vi "omni drive.vi"(0 "Drive RefNum":T3={"DevStatus"={"status"=FALSE, "code"=0, "source"=""}, "Motors[]"=[], "Square Inputs"=FALSE, "Max Output"=1.0}, 1 "X Axis":dbl, 2 "Y Axis":dbl, 3 "Z Axis":dbl, 4 "Drive Mode":T1=enum."Arcade Drive", 5 "Center Motor":T4={"DeviceStatus"={"status"=FALSE, "code"=0, "source"=""}, "Type"=enum."PWM", "PWM"={"Controller"=enum."Controller 1", "PWM Channel"=enum."Invalid", "DeadBand"={"Name"="", "maxPositivePwm"=0, "minPositivePwm"=0, "centerPwm"=0, "maxNegativePwm"=0, "minNegativePwm"=0, "angularRange"=0}}, "CAN"={"Device Number"=0, "Control Mode"=enum."Percent VBus", "Semaphore"=refnum, "Max Vout"=12.0, "TalonSRX Control Mode"=enum."Percent VBus"}, "Invert"=FALSE, "TransformRef"=refnum, "InvTransformRef"=refnum}) -> ()   [LabVIEW 2014]
uses:
  typedefs/omni drive mode.ctl
  <vilib>/Rock Robotics/WPI/RobotDrive/WPI_RobotDriveDevRef.ctl
  <vilib>/Rock Robotics/WPI/MotorControl/WPI_MotorControlDeviceRef.ctl
  <vilib>/Rock Robotics/WPI/MotorControl/WPI_MotorControlType.ctl
  <vilib>/Rock Robotics/SystemInterfaces/Typedef/FPGA_TypedefDigitalModule.ctl
  <vilib>/Rock Robotics/SystemInterfaces/DIO/FPGA_DIOPWMChannel.ctl
  <vilib>/Rock Robotics/WPI/PWM/WPI_PWMDeadband.ctl
  <vilib>/Rock Robotics/WPI/CAN/Jaguar/SubVIs/WPI_CANJaguar_ControlMode.ctl
  <vilib>/Rock Robotics/WPI/CAN/TalonSRX/WPI_CANTalonSRX_APIControlMode.ctl
  <vilib>/Rock Robotics/WPI/PWM/WPI_PWMTransform_ConPane.ctl
  global variables/devrefs.vi
  <vilib>/addons/control/pid/pid.llb/PID (DBL).vi
  <vilib>/Rock Robotics/WPI/RobotDrive/WPI_RobotDriveArcadeDrive_Standard(NoSaturation).vi
  global variables/dashboard data.vi
  <vilib>/addons/control/pid/NI_PID_pid.lvlib
panel:
  in  "Omni-Drive Tab Control":enum32{"Drive I/O", "PID", "Motor Controls"}(tab)
  in  "Spin Factor":dbl(slide) min=0.0 max=2.0 step=0.1 scale=0.0..2.0
  in  "PID Gains":T2={"proportional gain (Kc)"=0.003, "integral time (Ti, min)"=0.0012, "derivative time (Td, min)"=0.001} {"derivative time (Td, min)" step=0.0001 format="%.5f"; "integral time (Ti, min)" step=0.0001 format="%.5f"; "proportional gain (Kc)" step=0.0001 format="%.5f"}
  out "Gyro Temp °C":dbl
  out "Gyro Temp °F":dbl
  out "Setpoint Angle":dbl format="%#_6g°"
  out "Current Angle":dbl format="%#_g°"
  out "PID & Gyro Waveform Chart":cluster{"Angle":dbl, "output":dbl}(graph)
  out "Angular Rate":dbl
  # "Drive the Robot in Either Arcade Style or H-Drive Style"
  # "VI Inputs"
  # "OKish values rev1\nP: 0.00040\nI: 0.00100\nD: 0.00000\n\nPretty Good values\nP: 0.02\nI: 0.005\nD: 0.001\n\nBetter values?\nP: 0.0025\nI: 0.002\nD: 0.001"
  # "Thats a type def so you can't change it to the system\ncontrol otherwise it will no longer by linked to the typedef,\nand you can't re-link it"
  # "Temporary"
  # "Does this empty space make you feel uncomfortable?"
  # "Yes."
  # "I'm glad you feel that way."
  # "Note: Current Angle only updated in H-Drive, \nSetpoint updated in Arcade"
  # "°/sec"
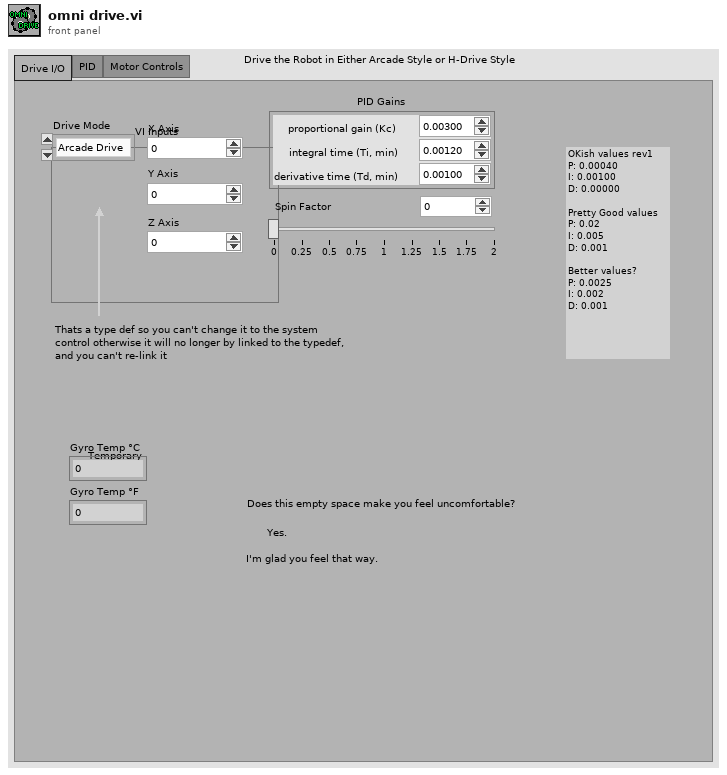
[diagram p1: front panel]
types:
  T1 = typedef "omni drive mode.ctl" = enum16{"Left/Right X/Y Control", "Arcade Drive", "H-Drive", "H-Drive Spin", "H-Drive PID", "Autonomous"}
  T2 = cluster{"proportional gain (Kc)":dbl, "integral time (Ti, min)":dbl, "derivative time (Td, min)":dbl}
  T3 = typedef "WPI_RobotDriveDevRef.ctl" = cluster{"DevStatus":errorcluster, "Motors[]":T4[], "Square Inputs":bool, "Max Output":dbl}
  T4 = typedef "WPI_MotorControlDeviceRef.ctl" = cluster{"DeviceStatus":errorcluster, "Type":T5, "PWM":cluster{"Controller":T6, "PWM Channel":T7, "DeadBand":T8}, "CAN":cluster{"Device Number":u8, "Control Mode":T9, "Semaphore":T10, "Max Vout":dbl, "TalonSRX Control Mode":T11}, "Invert":bool, "TransformRef":T12, "InvTransformRef":T12}
  T5 = typedef "WPI_MotorControlType.ctl" = enum16{"PWM", "CAN", "CANTalonSRX"}
  T6 = typedef "FPGA_TypedefDigitalModule.ctl" = enum16{"Controller 1"}
  T7 = typedef "FPGA_DIOPWMChannel.ctl" = enum8{"PWM 0", "PWM 1", "PWM 2", "PWM 3", "PWM 4", "PWM 5", "PWM 6", "PWM 7", "PWM 8", "PWM 9", "PWM MXP 0", "PWM MXP 1", "PWM MXP 2", "PWM MXP 3", "PWM MXP 4", "PWM MXP 5", "PWM MXP 6", "PWM MXP 7", "PWM MXP 8", "PWM MXP 9", "Invalid"}
  T8 = typedef "WPI_PWMDeadband.ctl" = cluster{"Name":string, "maxPositivePwm":i32, "minPositivePwm":i32, "centerPwm":i32, "maxNegativePwm":i32, "minNegativePwm":i32, "angularRange":u16}
  T9 = typedef "WPI_CANJaguar_ControlMode.ctl" = enum8{"Percent VBus", "Current", "Speed", "Position", "Voltage"}
  T10 = typedef "Semaphore RefNum" = refnum<k1>
  T11 = typedef "WPI_CANTalonSRX_APIControlMode.ctl" = enum8{"Percent VBus", "Speed", "Position", "Slave", "Unchanged / Invalid"}
  T12 = typedef "WPI_PWMTransform_ConPane.ctl" = refnum<vi>
  T13 = typedef "WPI_GyroDevRef.ctl" = cluster{"DevStatus":errorcluster, "Analog Module":T14, "Analog Channel":T15, "Offset":dbl, "Gain (VoltsPerDegree/Second)":dbl}
  T14 = typedef "FPGA_TypedefAnalogModule.ctl" = enum16{"Controller 1"}
  T15 = typedef "FPGA_AIChannel.ctl" = enum8{"AI 0", "AI 1", "AI 2", "AI 3", "AI MXP 0", "AI MXP 1", "AI MXP 2", "AI MXP 3", "Invalid"}
  T16 = typedef "WPI_EncoderDevRef.ctl" = cluster{"DevStatus":errorcluster, "EncoderIndex":T17, "CounterIndex":T18, "DistancePerCount":dbl, "Decoding Type":T19}
  T17 = typedef "FPGA_EncoderIdx.ctl" = enum8{"Enc 0", "Enc 1", "Enc 2", "Enc 3", "Enc 4", "Enc 5", "Enc 6", "Enc 7", "Invalid"}
  T18 = typedef "FPGA_CounterCtrSystemIndex.ctl" = enum8{"Ctr 0", "Ctr 1", "Ctr 2", "Ctr 3", "Ctr 4", "Ctr 5", "Ctr 6", "Ctr 7", "Invalid"}
  T19 = typedef "WPI_EncoderType.ctl" = enum16{"1x", "2x", "4x"}
  T20 = typedef "WPI_AnalogChannelDevRef.ctl" = cluster{"DevStatus":errorcluster, "Controller":T14, "Analog Channel":T15}
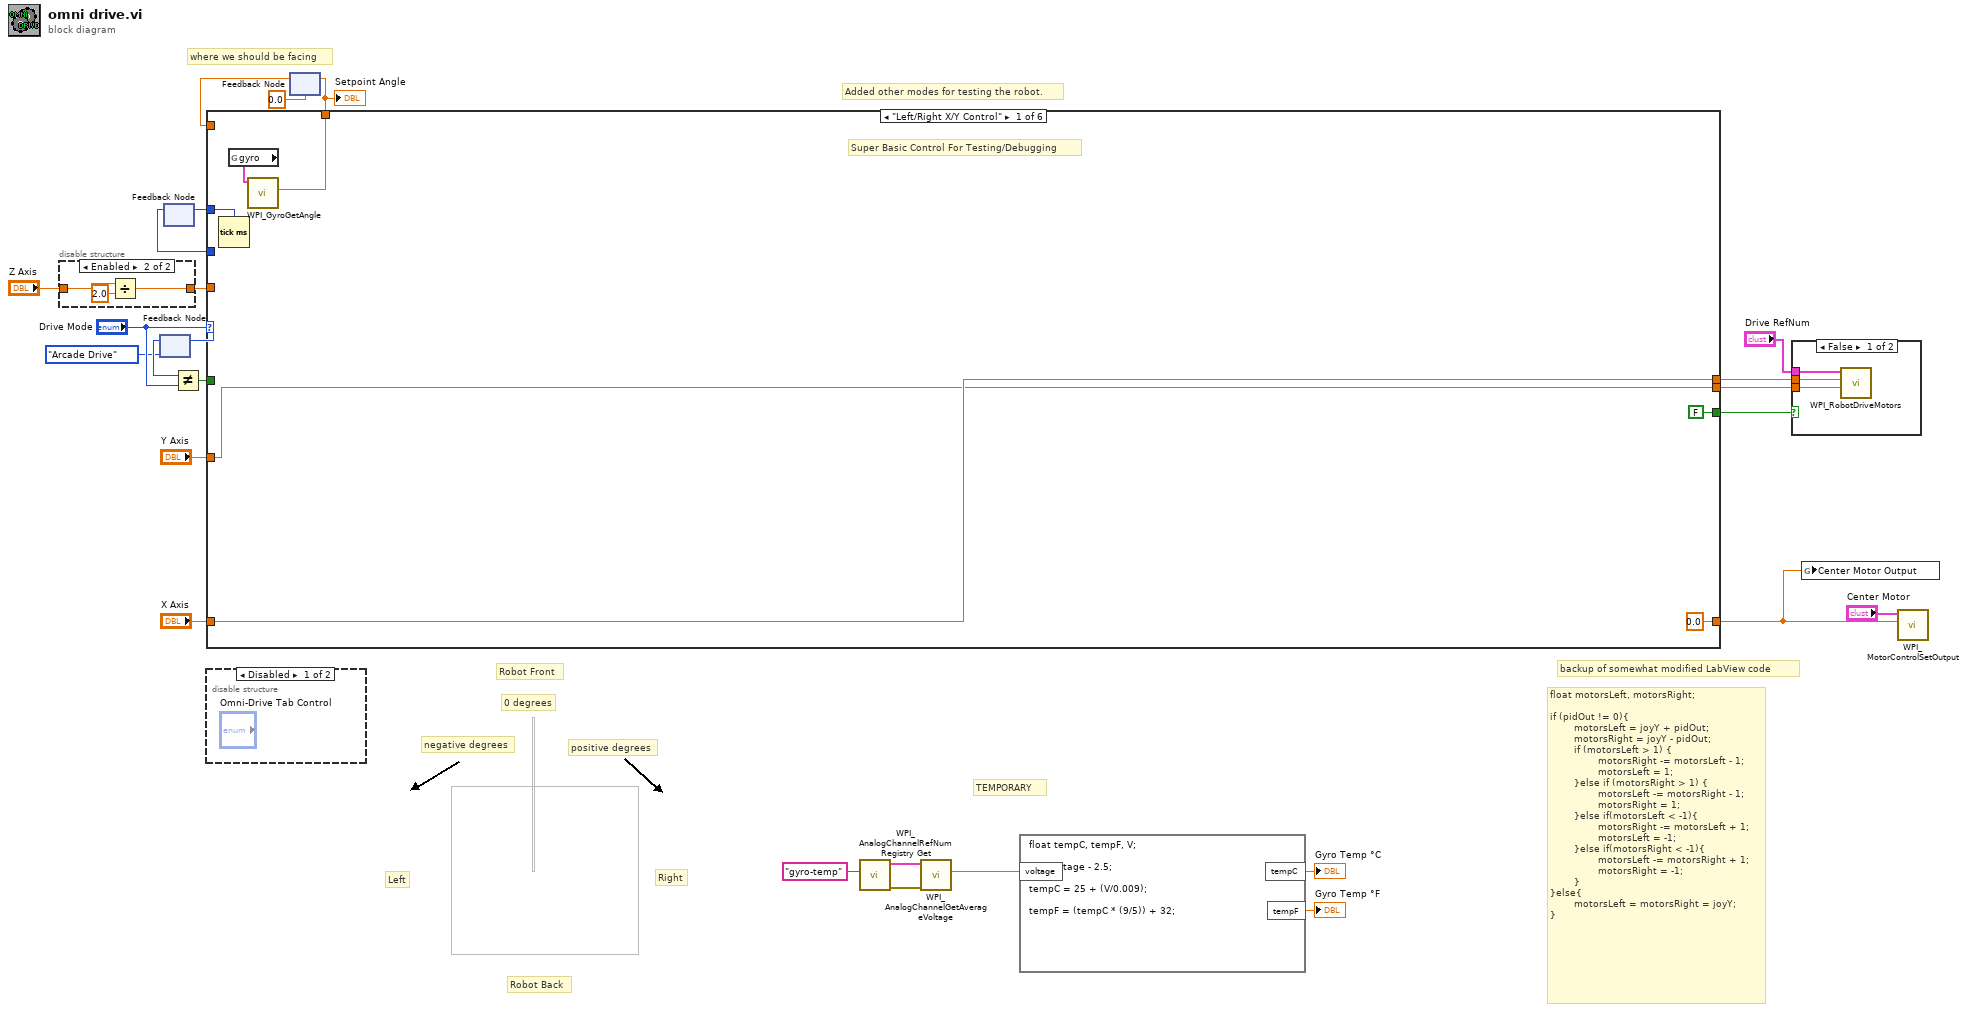
[diagram p0: block diagram]
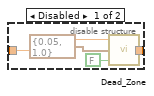
[diagram p2: hidden frame]
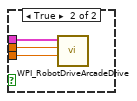
[diagram p4: hidden frame]
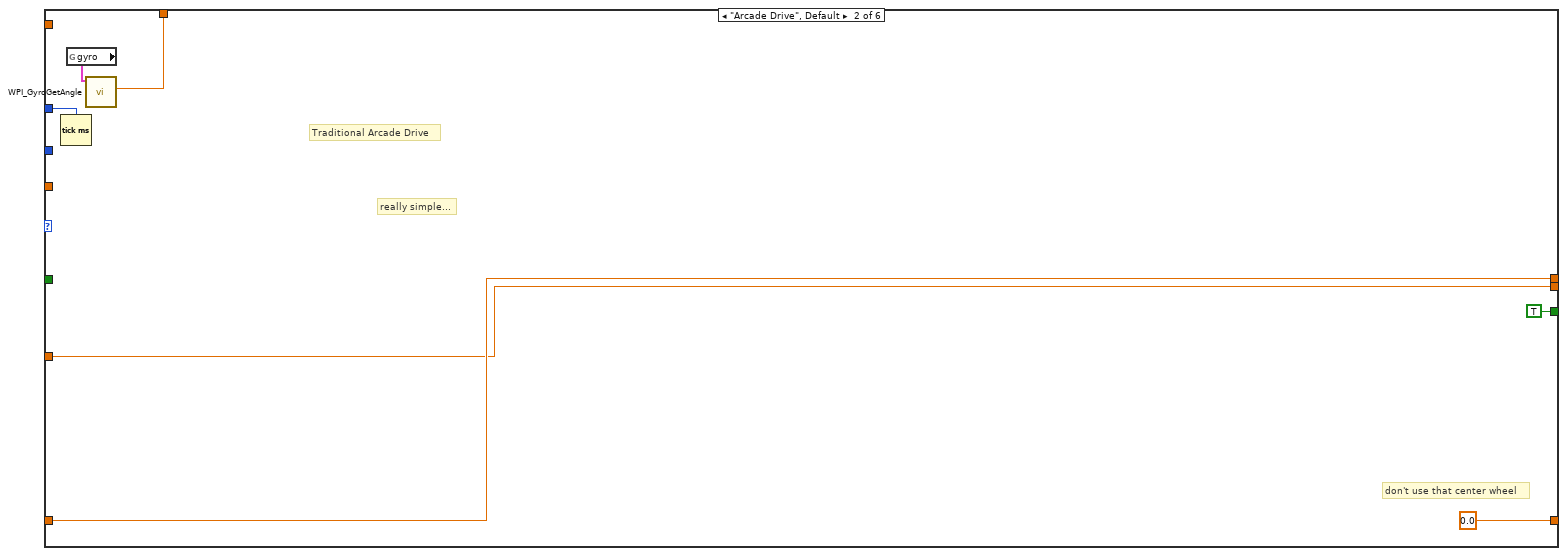
[diagram p5: hidden frame]
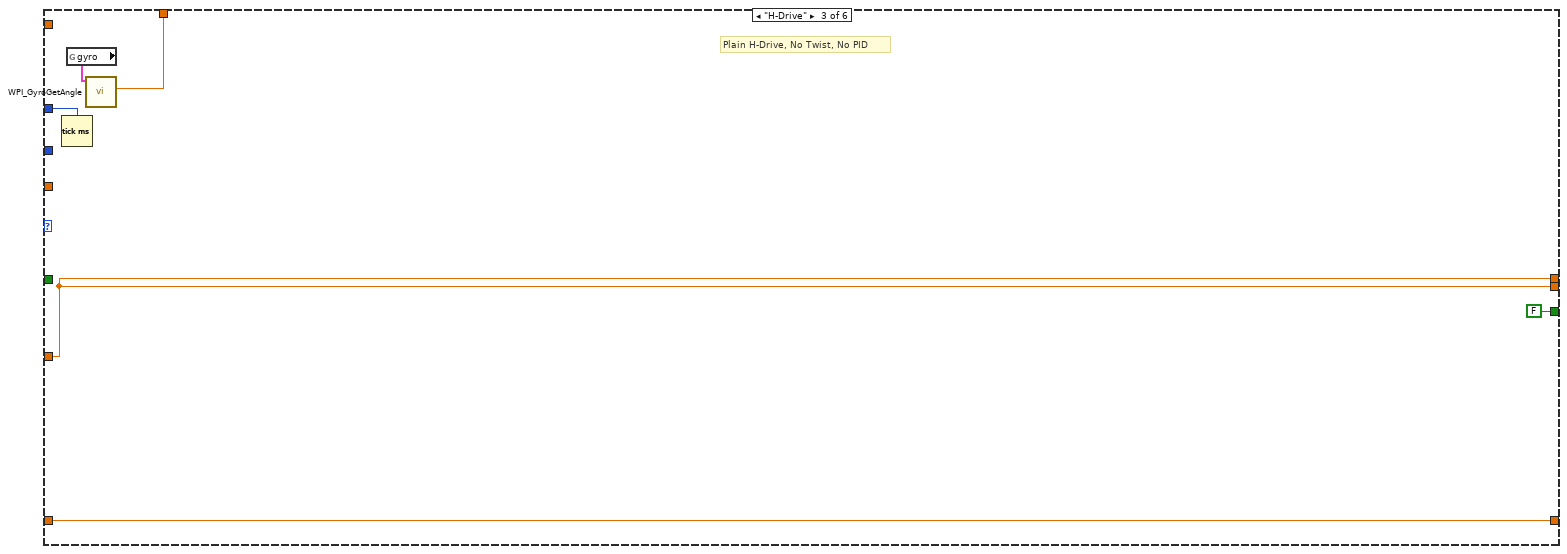
[diagram p6: hidden frame]
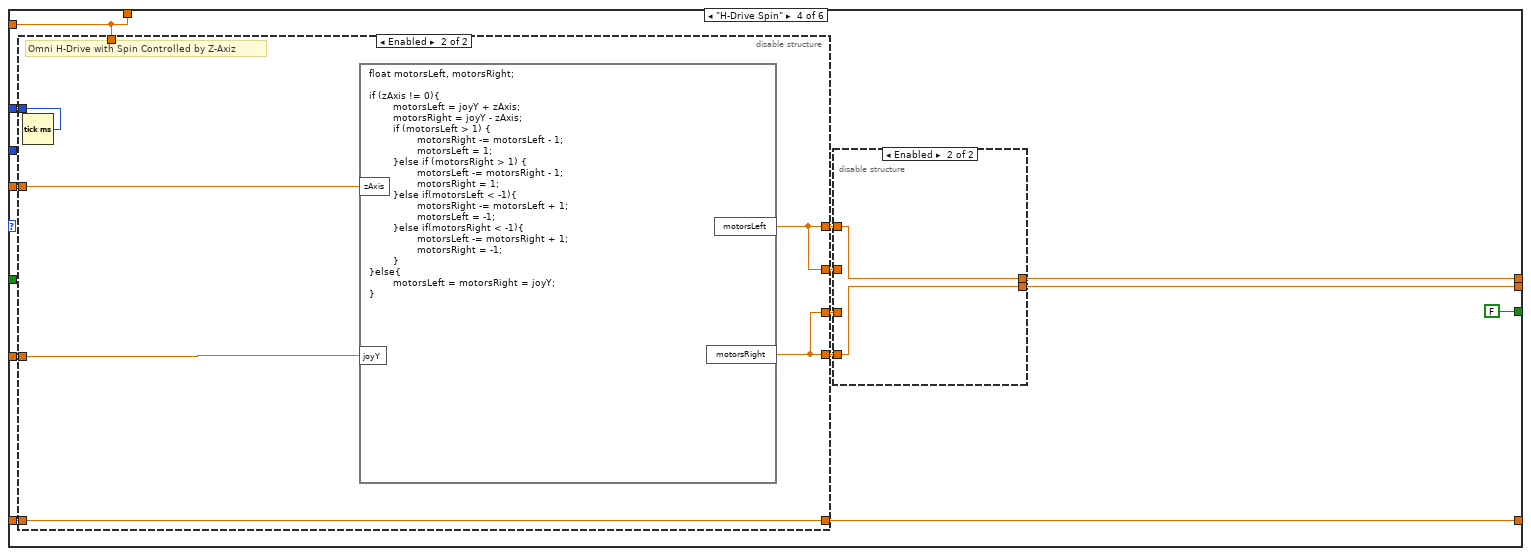
[diagram p7: hidden frame]
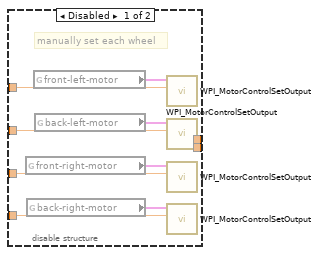
[diagram p8: hidden frame]
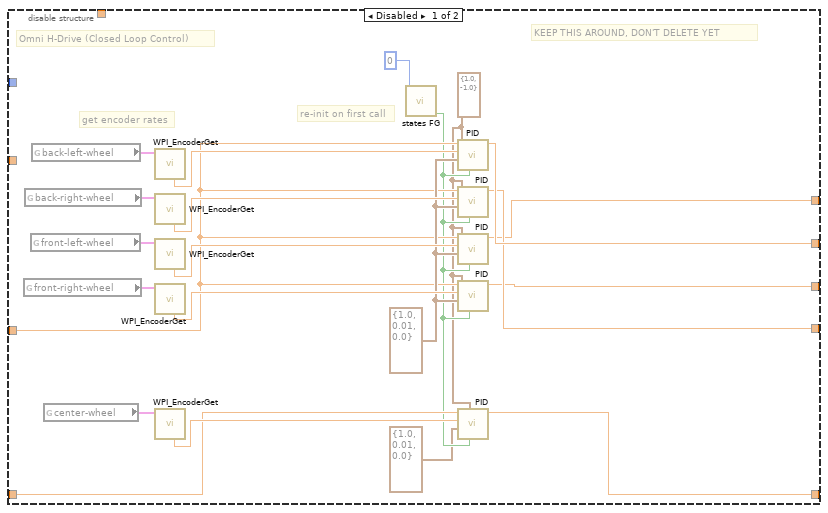
[diagram p9: hidden frame]
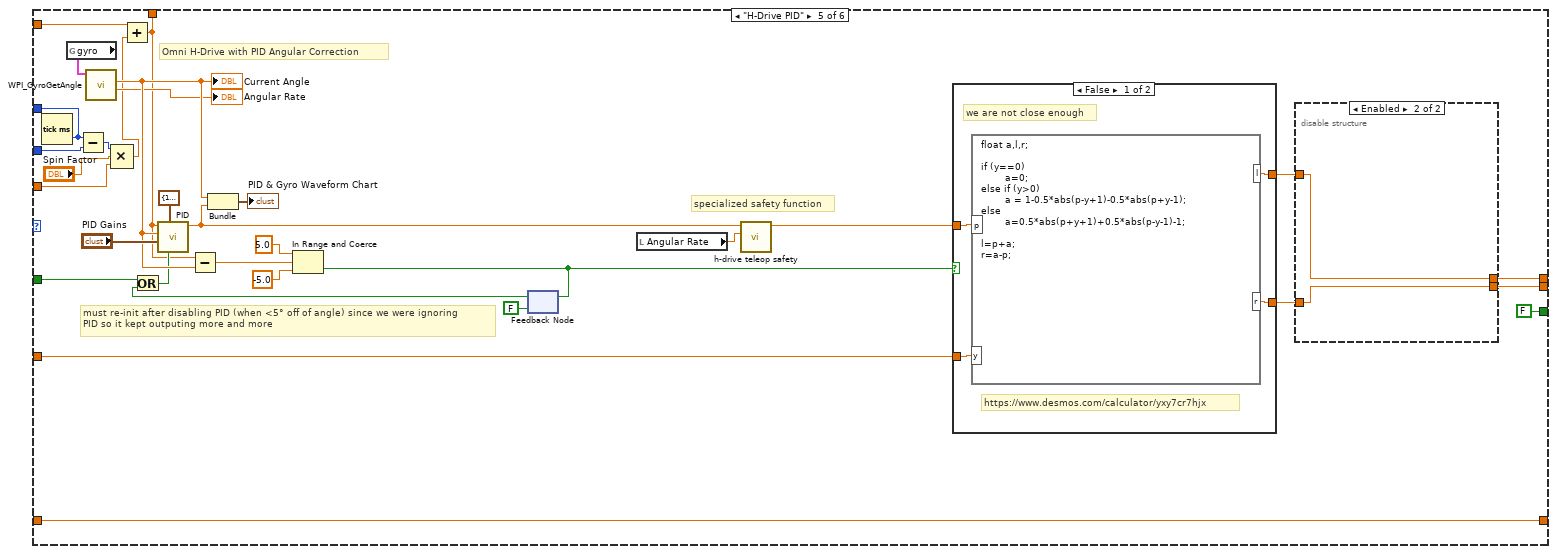
[diagram p10: hidden frame]
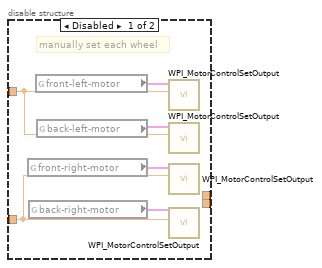
[diagram p11: hidden frame]
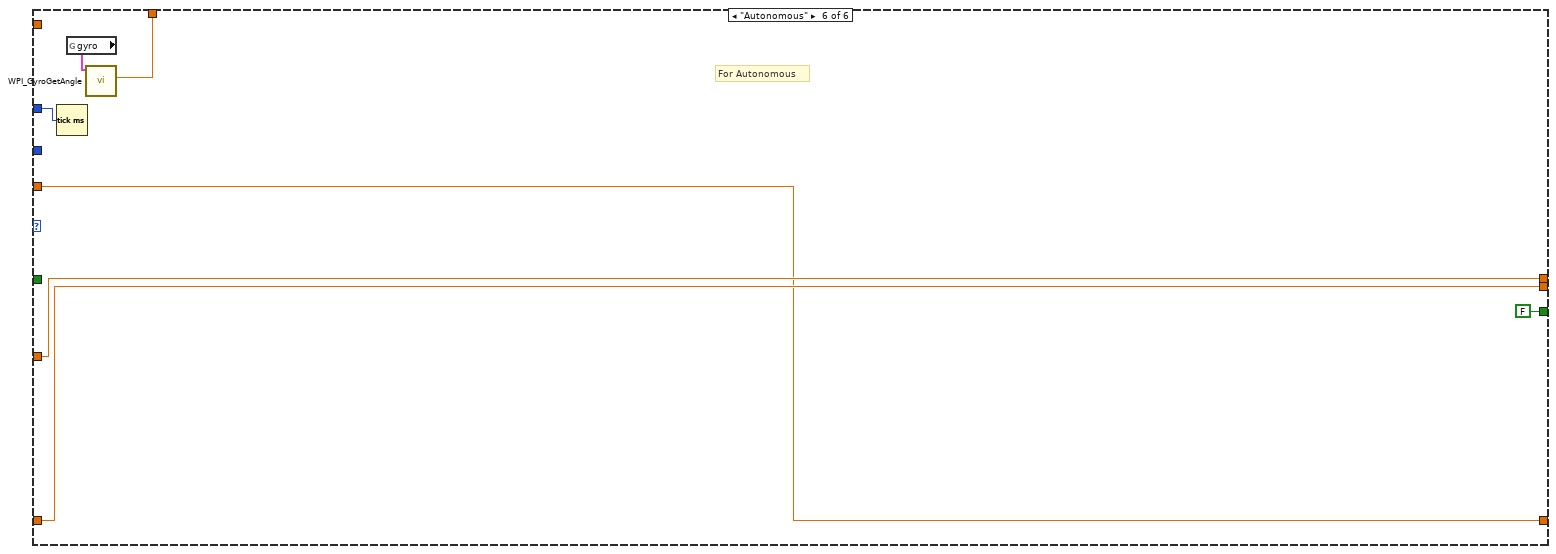
[diagram p13: hidden frame]
diagram:
  # "Added other modes for testing the robot."
  # "TEMPORARY"
  # "backup of somewhat modified LabView code"
  # "float motorsLeft, motorsRight;\n\nif (pidOut != 0){\n        motorsLeft = joyY + pidOut;\n        motorsRight = joyY - pidOut;\n        if (motorsLeft > 1) {\n                motorsRight -= motorsLeft - 1;\n                motorsLeft = 1;\n        }else if (motorsRight > 1) {\n                motorsLeft -= motorsRight - 1;\n                motorsRight = 1;\n        }else if(motorsLeft < -1){\n                motorsRight -= motorsLeft + 1;\n                motorsLeft = -1;\n        }else if(motorsRight < -1){\n                motorsLeft -= motorsRight + 1;\n                motorsRight = -1;\n        }\n}else{\n        motorsLeft = motorsRight = joyY;\n}"
  # "Robot Back"
  # "Right"
  # "Left"
  # "negative degrees"
  # "positive degrees"
  # "0 degrees"
  # "Robot Front"
  # "where we should be facing"
  n1 = disable-structure shown="Enabled" {
    disable-tunnel: [w29 w32] -> w2
    disable-tunnel: "Z Axis" -> [w28 w31]
    frame Disabled {
      n2 = call "Dead_Zone.vi"("Slope of 1"=FALSE, "Dead Zone and Limits"=cluster{dbl, dbl} {0.05, 1.0}, "Input"=w28) -> ("Output"=w29:dbl)  [unwired: 1 in]
    }
    frame Enabled {
      n3 = Divide(x=w31, y=2.0) -> (x/y=w32:dbl)
    }
  }
  n4 = feedback-in #1("Drive Mode") -> ()
  n5 = feedback #1(omni_drive_mode."Arcade Drive" ("Drive Mode")) -> (w18:T1)
  n6 = feedback #2() -> (w3:u32)  [unwired: 1 in]
  n7 = Not Equal?(x=w18, y="Drive Mode") -> (x != y?=w16:bool)
  n8 = disable-structure shown="Disabled" {
    frame Disabled {
    }
    frame Enabled {
    }
  }
  n9 = feedback #3(0.0) -> (w5:dbl)
  n10 = case shown="\"Left/Right X/Y Control\"" "Drive Mode" {
    tunnel: [0.0 ("X Axis") 0.0 w50 w62 w133 w152] -> w6
    tunnel: [w38 w45 w51 w54 w112 w153] -> w25
    tunnel: [w39 w46 w51 w55 w113 w155] -> w24
    tunnel: "X Axis" -> [w39 w46 w50 w63 w133 w153]
    tunnel: "Y Axis" -> [w38 w45 w51 w64 w134 w155]
    tunnel: [FALSE TRUE FALSE FALSE FALSE FALSE] -> w21
    tunnel: w16 -> [_ _ _ _ w132 _]
    tunnel: [w34 w43 w48 w61 w105 w150] -> w15
    tunnel: w5 -> [_ _ _ w61 w106 _]
    tunnel: w2 -> [_ _ _ w56 w108 w152]
    tunnel: [w33 w40 w47 w53 w111 w149] -> w4
    tunnel: w3 -> [_ _ _ _ w110 _]
    frame "Left/Right X/Y Control" {
      # "Super Basic Control For Testing/Debugging"
      n11 = Tick Count (ms)() -> (millisecond timer value=w33:u32)
      n12 = global read "devrefs.vi" "gyro"() -> (w35:T13)
      n13 = call <vilib>:"WPI_GyroGetAngle.vi"("GyroDevRef"=w35) -> ("Angle"=w34:dbl)  [unwired: 7 in, 3 out]
    }
    frame "Arcade Drive", Default {
      # "really simple..."
      # "don't use that center wheel"
      # "Traditional Arcade Drive"
      n14 = Tick Count (ms)() -> (millisecond timer value=w40:u32)
      n15 = global read "devrefs.vi" "gyro"() -> (w44:T13)
      n16 = call <vilib>:"WPI_GyroGetAngle.vi"("GyroDevRef"=w44) -> ("Angle"=w43:dbl)  [unwired: 7 in, 3 out]
    }
    frame "H-Drive" {
      # "Plain H-Drive, No Twist, No PID"
      n17 = Tick Count (ms)() -> (millisecond timer value=w47:u32)
      n18 = global read "devrefs.vi" "gyro"() -> (w49:T13)
      n19 = call <vilib>:"WPI_GyroGetAngle.vi"("GyroDevRef"=w49) -> ("Angle"=w48:dbl)  [unwired: 7 in, 3 out]
    }
    frame "H-Drive Spin" {
      n20 = disable-structure shown="Enabled" {
        disable-tunnel: w64 -> [w86 w103]
        disable-tunnel: w63 -> [w84 w102]
        disable-tunnel: [w80 w102] -> w62
        disable-tunnel: w61 -> [_ _]
        disable-tunnel: [w77 w101] -> w60
        disable-tunnel: [w79 w101] -> w59
        disable-tunnel: [w78 w100] -> w57
        disable-tunnel: [w76 w100] -> w58
        disable-tunnel: w56 -> [_ w98]
        disable-tunnel: [_ w99] -> w53
        frame Disabled {
          w87 = T2 {"proportional gain (Kc)"=1.0, "integral time (Ti, min)"=0.01, "derivative time (Td, min)"=0.0} ("PID gains")
          w82 = cluster{"output high":dbl, "output low":dbl} {"output high"=1.0, "output low"=-1.0} ("output range")
          # "KEEP THIS AROUND, DON'T DELETE YET"
          # "re-init on first call"
          # "get encoder rates"
          # "Omni H-Drive (Closed Loop Control)"
          n21 = global read "devrefs.vi" "front-right-wheel"() -> (w94:T16)
          n22 = global read "devrefs.vi" "back-right-wheel"() -> (w96:T16)
          n23 = global read "devrefs.vi" "front-left-wheel"() -> (w95:T16)
          n24 = global read "devrefs.vi" "back-left-wheel"() -> (w97:T16)
          n25 = global read "devrefs.vi" "center-wheel"() -> (w93:T16)
          n26 = call <vilib>:"WPI_EncoderGet.vi"("EncoderDevRef"=w97) -> ("Rate"=w91:dbl)  [unwired: 5 in, 5 out]
          n27 = call <vilib>:"WPI_EncoderGet.vi"("EncoderDevRef"=w96) -> ("Rate"=w90:dbl)  [unwired: 5 in, 5 out]
          n28 = call <vilib>:"WPI_EncoderGet.vi"("EncoderDevRef"=w95) -> ("Rate"=w89:dbl)  [unwired: 5 in, 5 out]
          n29 = call <vilib>:"WPI_EncoderGet.vi"("EncoderDevRef"=w94) -> ("Rate"=w88:dbl)  [unwired: 5 in, 5 out]
          n30 = call <vilib>:"WPI_EncoderGet.vi"("EncoderDevRef"=w93) -> ("Rate"=w85:dbl)  [unwired: 5 in, 5 out]
          n31 = call "states FG.vi"("Loop ID"=0) -> ("first call?"=w83:bool)  [unwired: 7 in, 3 out]
          n32 = call-poly <vilib>:"PID.vi"("reinitialize? (F)"=w83, "output range"=w82, "PID gains"=w87, "process variable"=w91, "setpoint"=w86) -> ("output"=w79:dbl)  [unwired: 5 in, 1 out]
          n33 = call-poly <vilib>:"PID.vi"("reinitialize? (F)"=w83, "output range"=w82, "PID gains"=w87, "process variable"=w90, "setpoint"=w86) -> ("output"=w78:dbl)  [unwired: 5 in, 1 out]
          n34 = call-poly <vilib>:"PID.vi"("reinitialize? (F)"=w83, "output range"=w82, "PID gains"=w87, "process variable"=w89, "setpoint"=w86) -> ("output"=w77:dbl)  [unwired: 5 in, 1 out]
          n35 = call-poly <vilib>:"PID.vi"("reinitialize? (F)"=w83, "output range"=w82, "PID gains"=w87, "process variable"=w88, "setpoint"=w86) -> ("output"=w76:dbl)  [unwired: 5 in, 1 out]
          n36 = call-poly <vilib>:"PID.vi"("reinitialize? (F)"=w83, "output range"=w82, "PID gains"=T2 {"proportional gain (Kc)"=1.0, "integral time (Ti, min)"=0.01, "derivative time (Td, min)"=0.0}, "process variable"=w85, "setpoint"=w84) -> ("output"=w80:dbl)  [unwired: 5 in, 1 out]
        }
        frame Enabled {
          # "Omni H-Drive with Spin Controlled by Z-Axiz"
          n37 = Tick Count (ms)() -> (millisecond timer value=w99:u32)
          n38 = formula code="float motorsLeft, motorsRight;\n\nif (zAxis != 0){\n        motorsLeft = joyY + zAxis;\n        motorsRight = joyY - zAxis;\n        if (motorsLeft > 1) {\n                motorsRight -= motorsLeft - 1;\n                motorsLeft = 1;\n        }else if (motorsRight > 1) {\n                motorsLeft -= motorsRight - 1;\n                motorsRight = 1;\n        }else if(motorsLeft < -1){\n                motorsRight -= motorsLeft + 1;\n                motorsLeft = -1;\n        }else if(motorsRight < -1){\n                motorsLeft -= motorsRight + 1;\n                motorsRight = -1;\n        }\n}else{\n        motorsLeft = motorsRight = joyY;\n}"("zAxis"=w98, "joyY"=w103) -> ("motorsLeft"=w101:dbl, "motorsRight"=w100:dbl)
        }
      }
      n39 = disable-structure shown="Enabled" {
        disable-tunnel: w60 -> [w69 w75]
        disable-tunnel: w59 -> [w68 _]
        disable-tunnel: w58 -> [w67 _]
        disable-tunnel: w57 -> [w66 w74]
        disable-tunnel: [_ w75] -> w55
        disable-tunnel: [_ w74] -> w54
        frame Disabled {
          # "manually set each wheel"
          n40 = global read "devrefs.vi" "front-right-motor"() -> (w70:T4)
          n41 = global read "devrefs.vi" "back-right-motor"() -> (w72:T4)
          n42 = global read "devrefs.vi" "front-left-motor"() -> (w71:T4)
          n43 = global read "devrefs.vi" "back-left-motor"() -> (w73:T4)
          n44 = call <vilib>:"WPI_MotorControlSetOutput.vi"("Output"=w69, "MotorControlDevRef"=w71) -> ()  [unwired: 7 in, 3 out]
          n45 = call <vilib>:"WPI_MotorControlSetOutput.vi"("Output"=w68, "MotorControlDevRef"=w73) -> ()  [unwired: 7 in, 3 out]
          n46 = call <vilib>:"WPI_MotorControlSetOutput.vi"("Output"=w67, "MotorControlDevRef"=w70) -> ()  [unwired: 7 in, 3 out]
          n47 = call <vilib>:"WPI_MotorControlSetOutput.vi"("Output"=w66, "MotorControlDevRef"=w72) -> ()  [unwired: 7 in, 3 out]
        }
        frame Enabled {
        }
      }
    }
    frame "H-Drive PID" {
      # "specialized safety function"
      # "must re-init after disabling PID (when <5° off of angle) since we were ignoring\nPID so it kept outputing more and more"
      # "Omni H-Drive with PID Angular Correction"
      n48 = Tick Count (ms)() -> (millisecond timer value=w111:u32)
      n49 = global read "devrefs.vi" "gyro"() -> (w128:T13)
      n50 = Subtract(x=w111, y=w110) -> (x-y=w109:u32)
      n51 = call <vilib>:"WPI_GyroGetAngle.vi"("GyroDevRef"=w128) -> ("Angular Rate"=→"Angular Rate":dbl, "Angle"=w125:dbl)  [unwired: 7 in, 2 out]
      "Current Angle" <- w125
      n52 = Compound Arithmetic op=MULTIPLY(w109, "Spin Factor", w108) -> (w104:dbl)
      n53 = Add(x=w106, y=w104) -> (x+y=w105:dbl)
      n54 = Subtract(x=w105, y=w125) -> (x-y=w121:dbl)
      n55 = In Range and Coerce(upper limit=5.0, x=w121, lower limit=-5.0 ("upper limit")) -> (In Range?=w124:bool)  [unwired: 1 out]
      n56 = feedback #4(FALSE) -> (w118:bool)
      n57 = Or(x=w132, y=w118) -> (x .or. y?=w123:bool)
      n58 = call-poly <vilib>:"PID.vi"("reinitialize? (F)"=w123, "output range"=cluster{"output high":dbl, "output low":dbl} {"output high"=1.0, "output low"=-1.0}, "PID gains"="PID Gains", "process variable"=w125, "setpoint"=w105) -> ("output"=w116:dbl)  [unwired: 5 in, 1 out]
      n59 = Bundle("Angle"=w125, "output"=w116) -> (→"PID & Gyro Waveform Chart":cluster{"Angle":dbl, "output":dbl})  [unwired: 1 in]
      n60 = feedback-in #4(w124) -> ()
      n61 = local read "Angular Rate"() -> (w114:dbl)
      n62 = call "h-drive teleop safety.vi"("Gyro Angular Rate"=w114, "Input"=w116) -> ("Output"=w115:dbl)  [unwired: 9 in]
      n63 = case shown="False" w124 {
        tunnel: w115 -> [w145 _]
        tunnel: w134 -> [w144 w148]
        tunnel: [w147 w148] -> w130
        tunnel: [w146 w148] -> w131
        frame False {
          # "https://www.desmos.com/calculator/yxy7cr7hjx"
          # "we are not close enough"
          n64 = formula code="float a,l,r;\n\nif (y==0) \n        a=0;\nelse if (y>0) \n        a = 1-0.5*abs(p-y+1)-0.5*abs(p+y-1);\nelse \n        a=0.5*abs(p+y+1)+0.5*abs(p-y-1)-1;\n\nl=p+a;\nr=a-p;"("p"=w145, "y"=w144) -> ("l"=w146:dbl, "r"=w147:dbl)
        }
        frame True {
          # "close enough... within 5°"
        }
      }
      n65 = disable-structure shown="Enabled" {
        disable-tunnel: w131 -> [w137 w143]
        disable-tunnel: w130 -> [w136 w142]
        disable-tunnel: [_ w143] -> w113
        disable-tunnel: [_ w142] -> w112
        frame Disabled {
          # "manually set each wheel"
          n66 = global read "devrefs.vi" "front-right-motor"() -> (w138:T4)
          n67 = global read "devrefs.vi" "back-right-motor"() -> (w140:T4)
          n68 = global read "devrefs.vi" "front-left-motor"() -> (w139:T4)
          n69 = global read "devrefs.vi" "back-left-motor"() -> (w141:T4)
          n70 = call <vilib>:"WPI_MotorControlSetOutput.vi"("Output"=w137, "MotorControlDevRef"=w139) -> ()  [unwired: 7 in, 3 out]
          n71 = call <vilib>:"WPI_MotorControlSetOutput.vi"("Output"=w137, "MotorControlDevRef"=w141) -> ()  [unwired: 7 in, 3 out]
          n72 = call <vilib>:"WPI_MotorControlSetOutput.vi"("Output"=w136, "MotorControlDevRef"=w138) -> ()  [unwired: 7 in, 3 out]
          n73 = call <vilib>:"WPI_MotorControlSetOutput.vi"("Output"=w136, "MotorControlDevRef"=w140) -> ()  [unwired: 7 in, 3 out]
        }
        frame Enabled {
        }
      }
    }
    frame "Autonomous" {
      # "For Autonomous"
      n74 = Tick Count (ms)() -> (millisecond timer value=w149:u32)
      n75 = global read "devrefs.vi" "gyro"() -> (w151:T13)
      n76 = call <vilib>:"WPI_GyroGetAngle.vi"("GyroDevRef"=w151) -> ("Angle"=w150:dbl)  [unwired: 7 in, 3 out]
    }
  }
  "Setpoint Angle" <- w15
  n77 = feedback-in #2(w4) -> ()
  n78 = feedback-in #3(w15) -> ()
  n79 = call <vilib>:"WPI_AnalogChannelRefNum Registry Get.vi"("refnum name"="gyro-temp") -> ("error out"=w12:errorcluster, "AIDeviceRef"=w11:T20)  [unwired: 9 in]
  n80 = call <vilib>:"WPI_AnalogChannelGetAverageVoltage.vi"("error in (no error)"=w12, "AIDeviceRef"=w11) -> ("Voltage"=w9:dbl)  [unwired: 7 in, 2 out]
  n81 = formula code="float tempC, tempF, V;\n\nV = voltage - 2.5;\n\ntempC = 25 + (V/0.009);\n\ntempF = (tempC * (9/5)) + 32;"("voltage"=w9) -> ("tempC"=→"Gyro Temp °C":dbl, "tempF"=→"Gyro Temp °F":dbl)
  n82 = case shown="False" w21 {
    tunnel: "Drive RefNum" -> [w158 w161]
    tunnel: w25 -> [w156 w160]
    tunnel: w24 -> [w157 w159]
    frame False {
      n83 = call <vilib>:"WPI_RobotDriveMotors.vi"("RightSpeed"=w156, "LeftSpeed"=w157, "RobotDriveDevRef"=w158) -> ()  [unwired: 6 in, 3 out]
    }
    frame True {
      n84 = call-poly <vilib>:"WPI_RobotDriveArcadeDrive.vi"("Y axis value"=w160, "X axis value"=w159, "RobotDriveDevRef"=w161) -> ()  [unwired: 6 in, 3 out]
    }
  }
  n85 = global write "dashboard data.vi" "Center Motor Output"(w6) -> ()
  n86 = call <vilib>:"WPI_MotorControlSetOutput.vi"("Output"=w6, "MotorControlDevRef"="Center Motor") -> ()  [unwired: 7 in, 3 out]
